vi "Create Offset Records.vi"(0 "Dataset Trans Id":T1) -> (2 "record":string)   [LabVIEW 2013]
uses:
  Global Data/Transactions/Dataset Transaction Id.ctl
  Global Data/Transactions/Dataset Source.ctl
  Global Data/Transactions/Dataset Type.ctl
  Apps/Yes No Button.ctl
  Data Access Objects/Metadata/DAO Actions.ctl
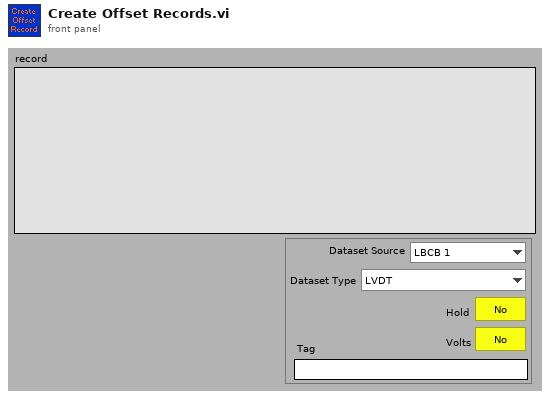
[diagram p1: front panel]
types:
  T1 = typedef "Dataset Transaction Id.ctl" = cluster{"Dataset Source":T2, "Dataset Type":T3, "Hold":T4, "Volts":T4, "Tag":string}
  T2 = typedef "Dataset Source.ctl" = enum16{"LBCB 1", "LBCB 2", "Combined", "External Sensors"}
  T3 = typedef "Dataset Type.ctl" = enum16{"LVDT", "Load Cell", "Actuator Command", "Servo Error", "Displacement Command", "Displacement", "Force"}
  T4 = typedef "Yes No Button.ctl" = bool
  T5 = typedef "DAO Actions.ctl" = enum16{"Init", "Get", "Set"}
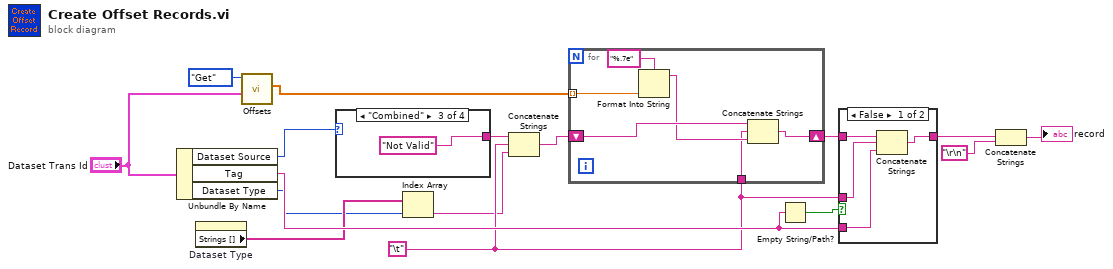
[diagram p0: block diagram]
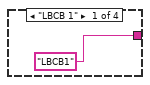
[diagram p3: hidden frame]
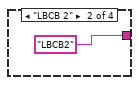
[diagram p4: hidden frame]
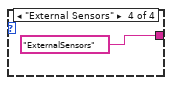
[diagram p5: hidden frame]
diagram:
  w2 = "\t"
  n1 = Unbundle By Name("Dataset Trans Id") -> ("Dataset Source"=w11:T2, "Tag"=w7:string, "Dataset Type"=w4:T3)
  n2 = property on="Dataset Type" class="Enum (strict)"() -> ("Strings []"=w5:string[])  [unwired: 2 in, 2 out]
  n3 = call "Offsets.vi"("Dataset Trans Id"="Dataset Trans Id", "DAO Actions"=DAO_Actions."Get") -> ("Data Out"=w13:dbl[])  [unwired: 7 in, 2 out]
  n4 = case shown="\"Combined\"" w11 {
    tunnel: ["LBCB1" "LBCB2" "Not Valid" "ExternalSensors"] -> w10
    frame "LBCB 1" {
    }
    frame "LBCB 2" {
    }
    frame "Combined" {
    }
    frame "External Sensors" {
    }
  }
  n5 = Index Array(array=w5, index=w4) -> (element=w1:string)
  n6 = Concatenate Strings(w10, w2, w1) -> (w3:string)
  n7 = for {
    shift-right: [w26] -> w9
    shift-left: w3 -> [w25]
    tunnel: w2 -> [w22]
    tunnel: w13 -> [w21] mode=indexing
    n8 = Format Into String(format string="%.7e", w21) -> (resulting string=w23:string)  [unwired: 2 in, 1 out]
    n9 = Concatenate Strings(w25, w22, w23) -> (w26:string)
  }
  n10 = Empty String/Path?(string/path=w7) -> (empty?=w8:bool)
  n11 = case shown="False" w8 {
    tunnel: w9 -> [w30 w31]
    tunnel: w7 -> [w28 _]
    tunnel: [w29 w31] -> w6
    tunnel: w2 -> [w27 _]
    frame False {
      n12 = Concatenate Strings(w30, w27, w28) -> (w29:string)
    }
    frame True {
    }
  }
  n13 = Concatenate Strings(w6, "\r\n") -> (→"record":string)
